vi "Extract Tabbed Control References.vi"(11 "Ctl Refnum":refnum<vi>) -> (3 "Control Map":T1(array[cluster]))   [LabVIEW 2023, in "Instruments.lvlib" / "Instruments.lvclass"]
uses:
  Library/Instruments.lvclass
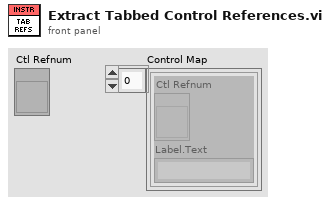
[diagram p1: front panel]
types:
  T1 = cluster{"Ctl Refnum":refnum<vi>, "Label.Text":string}[]
  T2 = cluster{"Ctl Refnum":refnum<vi>, "Label.Text":string}
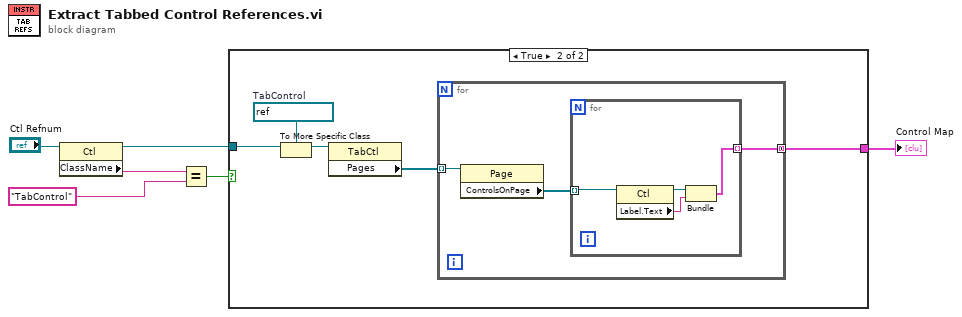
[diagram p0: block diagram]
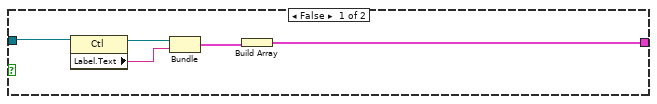
[diagram p2: hidden frame]
diagram:
  n1 = property class="Ctl"(reference="Ctl Refnum") -> (reference out=w5:refnum<vi>, "ClassName"=w2:string)  [unwired: 1 in, 1 out]
  n2 = Equal?(x=w2, y="TabControl") -> (x = y?=w4:bool)
  n3 = case shown="True" w4 {
    tunnel: w5 -> [w11 w16]
    tunnel: [w7 w12] -> w6
    frame False {
      n4 = property class="Ctl"(reference=w11) -> (reference out=w10:refnum<vi>, "Label.Text"=w9:string)  [unwired: 1 in, 1 out]
      n5 = Bundle("Ctl Refnum"=w10, "Label.Text"=w9) -> (w8:T2)  [unwired: 1 in]
      n6 = Build Array(w8) -> (w7:T1)
    }
    frame True {
      w15 = refnum<vi> refnum  # TabControl
      n7 = To More Specific Class(target class=w15, reference=w16) -> (specific class reference=w14:refnum<vi>)  [unwired: 1 in, 1 out]
      n8 = property class="TabCtl"(reference=w14) -> ("Pages"=w13:refnum<vi>[])  [unwired: 1 in, 2 out]
      n9 = for {
        tunnel: w13 -> [w19] mode=indexing
        tunnel: [w17] -> w12 mode=concatenating
        n10 = property class="Page"(reference=w19) -> ("ControlsOnPage"=w18:refnum<vi>[])  [unwired: 1 in, 2 out]
        n11 = for {
          tunnel: w18 -> [w23] mode=indexing
          tunnel: [w20] -> w17 mode=indexing
          n12 = property class="Ctl"(reference=w23) -> (reference out=w21:refnum<vi>, "Label.Text"=w22:string)  [unwired: 1 in, 1 out]
          n13 = Bundle(w21, "Label.Text"=w22) -> (w20:cluster{refnum<vi>, "Label.Text":string})  [unwired: 1 in]
        }
      }
    }
  }
  "Control Map" <- w6
